vi "Write Column Header.vi"(8 "error in (no error)":errorcluster, 10 "Column Header":string, 11 "Generic Data Type in":refnum<class "Generic Data Type.lvclass">) -> (0 "error out":errorcluster, 3 "Generic Data Type out":refnum<class "Generic Data Type.lvclass">)   [LabVIEW 2018, in "Generic Data Type.lvclass"]
uses:
  Generic Data Type.lvclass
  Generic Data Type.lvclass/Generic Data Type.ctl
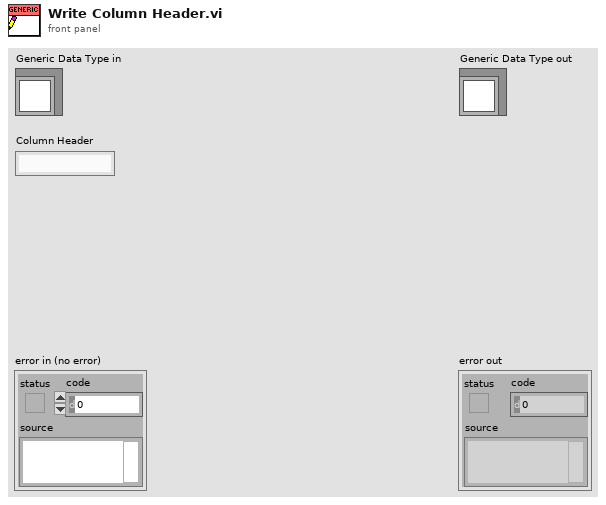
[diagram p1: front panel]
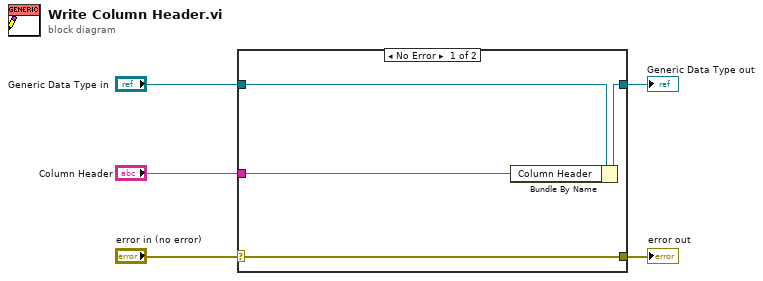
[diagram p0: block diagram]
diagram:
  n1 = case shown="No Error" "error in (no error)" {
    selector: "error in (no error)" -> [w9 w10]
    tunnel: [w9 w10] -> w4
    tunnel: [w7 w11] -> w2
    tunnel: "Generic Data Type in" -> [w8 w11]
    tunnel: "Column Header" -> [w6 _]
    frame No Error {
      n2 = Bundle By Name(cluster=w8, "Column Header"=w6) -> (w7:refnum<class "Generic Data Type.lvclass">)
    }
    frame Error {
    }
  }
  "error out" <- w4
  "Generic Data Type out" <- w2
